vi "SwerveDriveLogic.vi"(9 "Speeds":dbl[](array[numeric]), 10 "AngleSetpoints":dbl[](array[numeric]), 11 "AngleEncoders":dbl[](array[numeric])) -> (2 "AngleMotorsReversed":bool[](array[boolean]), 3 "AngleMotorOutputs":dbl[](array[numeric]))   [LabVIEW 2018]
uses:
  <vilib>/Rock Robotics/Network Tables/NT Write Numeric Array.vi
  <vilib>/addons/control/pid/pid.llb/PID (DBL).vi
  <vilib>/Rock Robotics/Network Tables/NT Write Boolean Array.vi
  <vilib>/addons/control/pid/NI_PID_pid.lvlib
panel:
  out "Back right module":dbl(knob)
  out "Back left module":dbl(knob)
  out "Front left module":dbl(knob)
  out "Front right module":dbl(knob)
  in  "PID gains":T1={"proportional gain (Kc)"=0.05, "integral time (Ti, min)"=0.0, "derivative time (Td, min)"=0.0} {"derivative time (Td, min)" format="%.15f"; "integral time (Ti, min)" format="%.3f"; "proportional gain (Kc)" format="%.3f"}
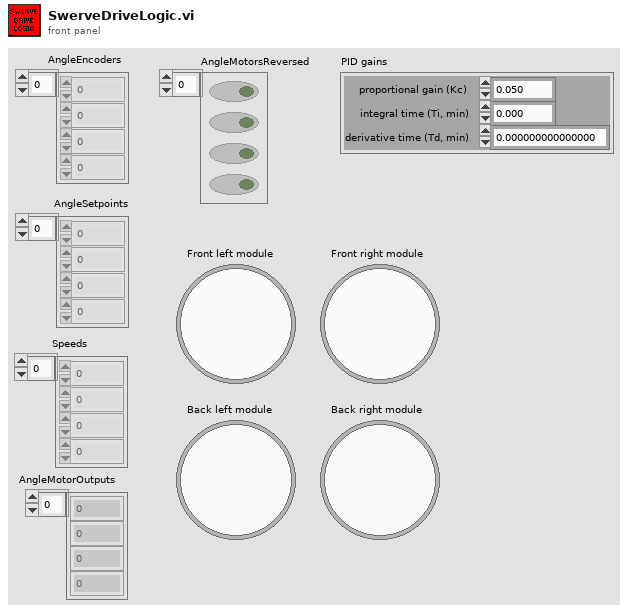
[diagram p1: front panel]
types:
  T1 = cluster{"proportional gain (Kc)":dbl, "integral time (Ti, min)":dbl, "derivative time (Td, min)":dbl}
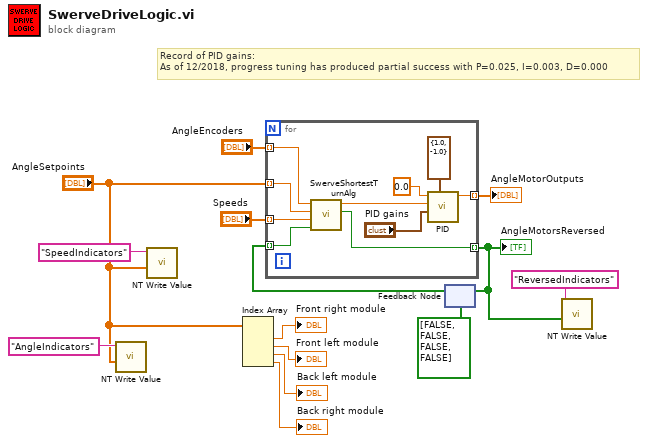
[diagram p0: block diagram]
diagram:
  # "Record of PID gains:\nAs of 12/2018, progress tuning has produced partial success with P=0.025, I=0.003, D=0.000"
  n1 = call-poly <vilib>:"NT Write Value.vi"("Numeric Array"="AngleSetpoints", "Name"="AngleIndicators") -> ()  [unwired: 9 in, 1 out]
  n2 = call-poly <vilib>:"NT Write Value.vi"("Numeric Array"="AngleSetpoints", "Name"="SpeedIndicators") -> ()  [unwired: 9 in, 1 out]
  n3 = Index Array(array="AngleSetpoints") -> (element #1=→"Front right module":dbl, element #2=→"Front left module":dbl, element #3=→"Back left module":dbl, element #4=→"Back right module":dbl)  [unwired: 4 in]
  n4 = feedback #1(bool[] [FALSE, FALSE, FALSE, FALSE] ("SwerveMotorsFlipped")) -> (w13:bool[])
  n5 = for {
    tunnel: "AngleEncoders" -> [w15] mode=indexing
    tunnel: "Speeds" -> [w22] mode=indexing
    tunnel: w13 -> [w18] mode=indexing
    tunnel: "AngleSetpoints" -> [w17] mode=indexing
    tunnel: [w21] -> w11 mode=indexing
    tunnel: [w20] -> w2 mode=indexing
    n6 = call "SwerveShortestTurnAlg.vi"("SwerveMotorsFlipped?"=w18, "SwerveSpeed"=w22, "AngleSetpoint"=w17, "AngleEncoder"=w15) -> ("FlipSwerveMotors"=w20:bool, "PIDInput"=w16:dbl)  [unwired: 6 in]
    n7 = call-poly <vilib>:"PID.vi"("output range"=cluster{"output high":dbl, "output low":dbl} {"output high"=1.0, "output low"=-1.0}, "PID gains"="PID gains", "process variable"=w16, "setpoint"=0.0) -> ("output"=w21:dbl)  [unwired: 6 in, 1 out]
  }
  "AngleMotorOutputs" <- w11
  "AngleMotorsReversed" <- w2
  n8 = feedback-in #1(w2) -> ()
  n9 = call-poly <vilib>:"NT Write Value.vi"("Boolean Array"=w2, "Name"="ReversedIndicators") -> ()  [unwired: 9 in, 1 out]
